vi "Host-Echo-Test.vi"() -> ()   [LabVIEW 2015]
uses:
  <vilib>/rvi/interface/RandomDataEmulation/nirviRandomDataOpen.vi
  <vilib>/rvi/interface/RandomDataEmulation/nirviRandomDataDMAMethods.vi
  <vilib>/rvi/interface/RandomDataEmulation/nirviRandomDataClose.vi
  <vilib>/rvi/interface/nirviOpenFPGA/nirviOpenFPGA.xnode
  Fpga-Version/PXI-7953R/Benchmarking/Echo-Test.vi
  <vilib>/rvi/interface/nirviMethod/nirviMethod.xnode
  <vilib>/rvi/interface/nirviCloseFPGA/nirviCloseFPGA.xnode
panel:
  out "Numeric":i32
  out "Packets sent":i32
  out "Elements Read":i32
  out "Elements Remaining":u32
  out "error out":errorcluster
  in  "error in":errorcluster
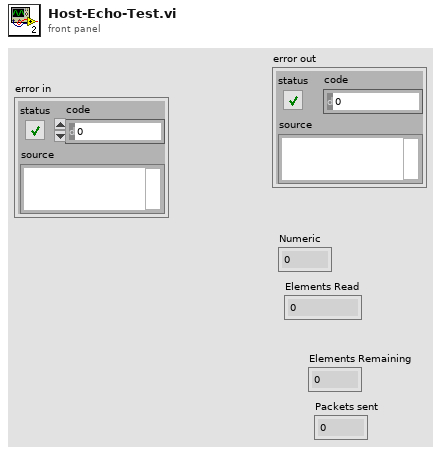
[diagram p1: front panel]
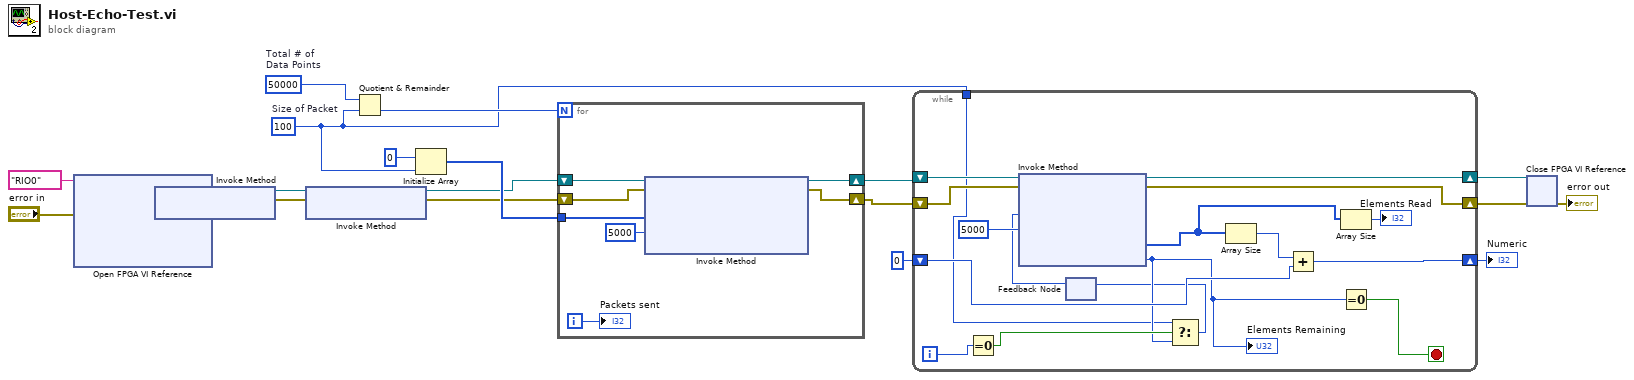
[diagram p0: block diagram]
diagram:
  w3 = 100  # Size of Packet
  w17 = 50000  # Total # of Data Points
  n1 = xnode "Open FPGA VI Reference"("error in"="error in", "resource name"=tag "RIO0") -> ("FPGA VI Reference Out"=w20:refnum<k20>, "error out"=w19:errorcluster)
  n2 = xnode "Invoke Method"("FPGA VI Reference In"=w20, "error in"=w19) -> ("FPGA VI Reference Out"=w7:refnum<k20>, "error out"=w6:errorcluster)
  n3 = xnode "Invoke Method"("FPGA VI Reference In"=w7, "error in"=w6) -> ("FPGA VI Reference Out"=w4:refnum<k20>, "error out"=w5:errorcluster)
  n4 = Quotient & Remainder(x=w17, y=w3) -> (floor(x/y)=w16:i32)  [unwired: 1 out]
  n5 = Initialize Array(u64 0, w3) -> (w8:u64[])
  n6 = for {
    N: w16 -> [_]
    tunnel: w8 -> [w27]
    shift-right: [w25] -> w14
    shift-left: w4 -> [w24]
    shift-right: [w22] -> w13
    shift-left: w5 -> [w23]
    i -> [w21]
    n7 = xnode "Invoke Method"("FPGA VI Reference In"=w24, "error in"=w23, "Data"=w27, "Timeout (ms)"=5000) -> ("FPGA VI Reference Out"=w25:refnum<k20>, "error out"=w22:errorcluster)  [unwired: 1 out]
    "Packets sent" <- w21
  }
  n8 = while {
    shift-right: [w42] -> w12
    shift-left: w14 -> [w40]
    shift-right: [w41] -> w11
    shift-left: w13 -> [w39]
    tunnel: w3 -> [w30]
    shift-right: [w36] -> w2
    shift-left: 0 -> [w35]
    i -> [w33]
    stop <- w43 stop-if-true
    n9 = Equal To 0?(x=w33) -> (x = 0?=w32:bool)
    n10 = feedback #1() -> (w28:u32)  [unwired: 1 in]
    n11 = xnode "Invoke Method"("FPGA VI Reference In"=w40, "error in"=w39, "Number of Elements"=w28, "Timeout (ms)"=5000) -> ("FPGA VI Reference Out"=w42:refnum<k20>, "error out"=w41:errorcluster, "Data"=w34:u64[], "Elements Remaining"=w31:u32)
    "Elements Remaining" <- w31
    n12 = Select(t=w30, s=w32, f=w31) -> (s? t:f=w29:u32)
    n13 = feedback-in #1(w29) -> ()
    n14 = Array Size(array=w34) -> (size(s)=w37:i32)
    n15 = Add(x=w37, y=w35) -> (x+y=w36:i32)
    n16 = Array Size(array=w34) -> (size(s)=→"Elements Read":i32)
    n17 = Equal To 0?(x=w31) -> (x = 0?=w43:bool)
  }
  "Numeric" <- w2
  n18 = xnode "Close FPGA VI Reference"("FPGA VI Reference In"=w12, "error in"=w11) -> ("error out"=→"error out":errorcluster)
